vi "RobotStateLookUp(SubVI).vi"(11 "Numeric":u8) -> (3 "element":string)   [LabVIEW 2013]
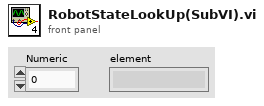
[diagram p1: front panel]
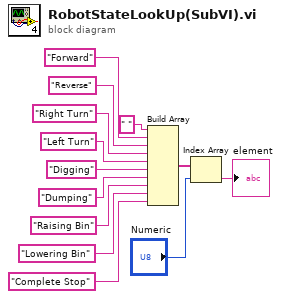
[diagram p0: block diagram]
diagram:
  n1 = Build Array(" " ("element"), "Forward", "Reverse", "Right Turn", "Left Turn", "Digging", "Dumping", "Raising Bin", "Lowering Bin", "Complete Stop") -> (w11:string[])
  n2 = Index Array(array=w11, index="Numeric") -> (element=→"element":string)
